vi "patterns_rectangular_grid.vi"(1 "spacing/m":dbl=2.0, 2 "N":cluster{i32, i32}) -> (0 "Spots":T1[](array[typedef]) {"Amplitude Correction" step=0.1; "Line Trapping"."Phase Gradient" step=0.05; "Line Trapping"."Vector"."x" step=1e-06 format="%#_6p"; "Line Trapping"."Vector"."y" step=1e-06 format="%#_6p"; "Line Trapping"."Vector"."z" step=1e-06 format="%#_6p"; "NA Position"."r" step=1e-06; "NA Position"."y" step=1e-06; "NA Position"."x" step=1e-06; "Position"."z" step=1e-06; "Position"."y" step=1e-06; "Position"."x" step=1e-06; "Phase" step=0.7753; "Intensity" step=0.1})   [LabVIEW 2015]
uses:
  spot.ctl
  line_trapping.ctl
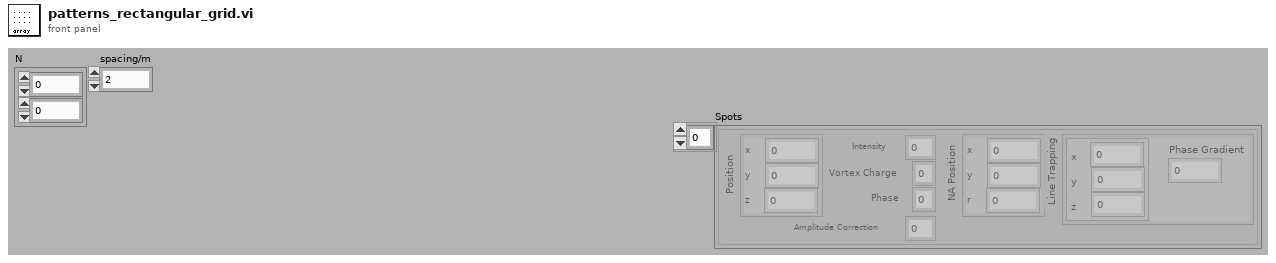
[diagram p1: front panel]
types:
  T1 = typedef "spot.ctl" = cluster{"Position":cluster{"x":dbl, "y":dbl, "z":dbl}, "Intensity":dbl, "Vortex Charge":i8, "Phase":dbl, "NA Position":cluster{"x":dbl, "y":dbl, "r":dbl}, "Line Trapping":T2, "Amplitude Correction":dbl}
  T2 = typedef "line_trapping.ctl" = cluster{"Vector":cluster{"x":dbl, "y":dbl, "z":dbl}, "Phase Gradient":dbl}
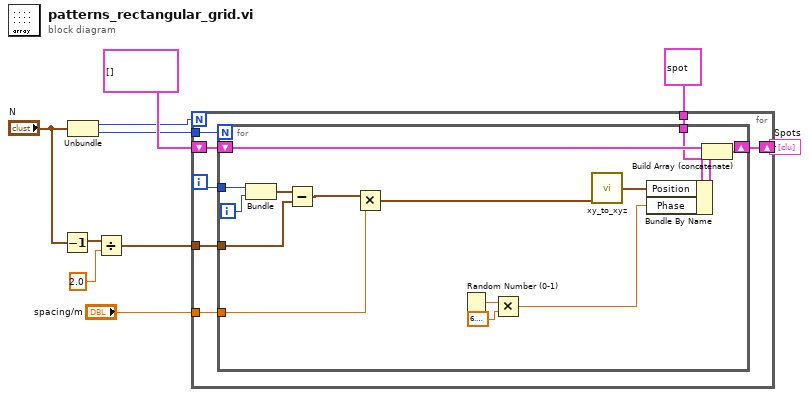
[diagram p0: block diagram]
diagram:
  n1 = Decrement(x="N") -> (x-1=w4:cluster{i32, i32})
  n2 = Unbundle("N") -> (w7:i32, w6:i32)
  n3 = Divide(x=w4, y=2.0 ("x*y")) -> (x/y=w2:cluster{dbl, dbl})
  n4 = for {
    N: w7 -> [_]
    shift-right: [w15] -> w9
    shift-left: T1[] [] ("Spots 2") -> [w16]
    tunnel: T1 {"Position"={"x"=0.0, "y"=0.0, "z"=0.0}, "Intensity"=1.0, "Vortex Charge"=0, "Phase"=0.0, "NA Position"={"x"=0.0, "y"=0.0, "r"=1.0}, "Line Trapping"={"Vector"={"x"=0.0, "y"=0.0, "z"=0.0}, "Phase Gradient"=0.0}, "Amplitude Correction"=0.0} ("element") -> [w14]
    tunnel: w6 -> [w13]
    tunnel: w2 -> [w12]
    tunnel: "spacing/m" -> [w11]
    i -> [w17]
    n5 = for {
      N: w13 -> [_]
      tunnel: w17 -> [w24]
      shift-right: [w32] -> w15
      shift-left: w16 -> [w31]
      tunnel: w14 -> [w29]
      tunnel: w12 -> [w21]
      tunnel: w11 -> [w19]
      i -> [w23]
      n6 = Bundle(w24, w23) -> (w22:cluster{i32, i32})  [unwired: 1 in]
      n7 = Subtract(x=w22, y=w21) -> (x-y=w20:cluster{dbl, dbl})
      n8 = Multiply(x=w20, y=w19) -> (x*y=w18:cluster{dbl, dbl})
      n9 = Random Number (0-1)() -> (number: 0 to 1=w28:dbl)
      n10 = Multiply(x=w28, y=6.283185307179586) -> (x*y=w26:dbl)
      n11 = call "xy_to_xyz.vi"("Position (2D)"=w18) -> ("Position (3D)"=w25:cluster{dbl, dbl, dbl})  [unwired: 3 in]
      n12 = Bundle By Name(cluster=w29, "Position"=w25, "Phase"=w26) -> (w30:T1)
      n13 = Build Array (concatenate)(w31, w30) -> (w32:T1[])
    }
  }
  "Spots" <- w9
